vi "Error Word Bits Checker.vi"(6 "error text in":string, 8 "error in":errorcluster, 9 "number of bits":i32, 10 "start bit":i32, 11 "reserved bits in":bool[](array[boolean])=[TRUE, TRUE, TRUE, TRUE, TRUE, TRUE, TRUE, TRUE, FALSE, FALSE, FALSE, FALSE, FALSE, FALSE, FALSE, FALSE, FALSE, FALSE, FALSE, FALSE, FALSE, FALSE, FALSE, FALSE, FALSE, FALSE, FALSE, FALSE, FALSE, FALSE, FALSE, TRUE]) -> (0 "error out":errorcluster, 3 "reserved bits out":bool[](array[boolean]))   [LabVIEW 2020, in "ARINC 429 Import.lvlib"]
uses:
  ARINC 429 Import.lvlib
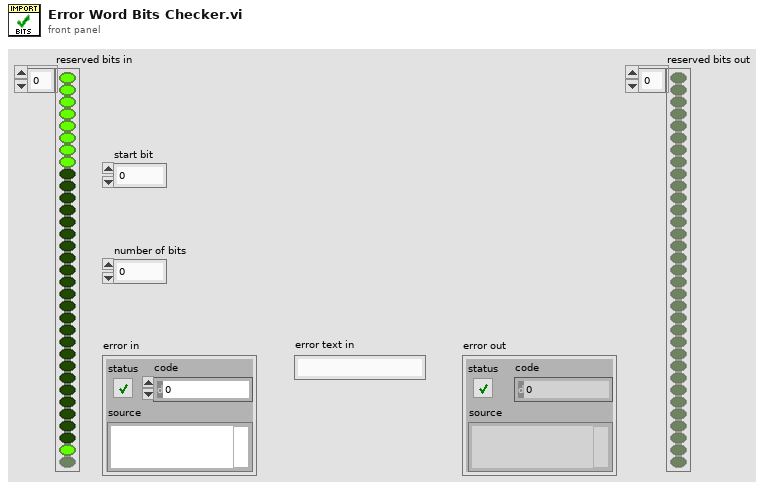
[diagram p1: front panel]
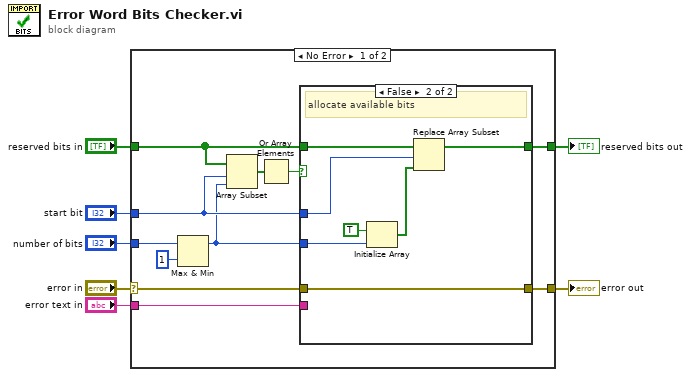
[diagram p0: block diagram]
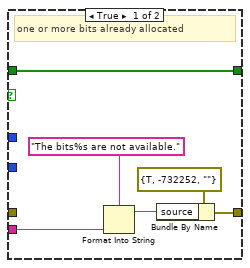
[diagram p2: hidden frame]
diagram:
  n1 = case shown="No Error" "error in" {
    selector: "error in" -> [w14 w33]
    tunnel: "start bit" -> [w18 _]
    tunnel: "number of bits" -> [w17 _]
    tunnel: [w15 w33] -> w4
    tunnel: "error text in" -> [w16 _]
    tunnel: "reserved bits in" -> [w13 w32]
    tunnel: [w8 w32] -> w1
    frame No Error {
      n2 = Max & Min(x=w17, y=1) -> (max(x,y)=w9:i32)  [unwired: 1 out]
      n3 = Array Subset(array=w13, index=w18, length=w9) -> (w12:bool[])
      n4 = Or Array Elements(Boolean array=w12) -> (logical OR=w11:bool)
      n5 = case shown="False" w11 {
        tunnel: [w24 w31] -> w8
        tunnel: w13 -> [w24 w30]
        tunnel: w9 -> [_ w29]
        tunnel: w18 -> [_ w26]
        tunnel: w16 -> [w20 _]
        tunnel: [w19 w25] -> w15
        tunnel: w14 -> [_ w25]
        frame True {
          # "one or more bits already allocated"
          n6 = Format Into String(format string="The bits%s are not available." ("source"), w20) -> (resulting string=w23:string)  [unwired: 2 in, 1 out]
          n7 = Bundle By Name(cluster=errorcluster {"status"=TRUE, "code"=-732252, "source"=""} ("error constant"), "source"=w23) -> (w19:errorcluster)
        }
        frame False {
          # "allocate available bits"
          n8 = Initialize Array(TRUE, w29) -> (w27:bool[])
          n9 = Replace Array Subset(array=w30, new element=w27, index=w26) -> (w31:bool[])
        }
      }
    }
    frame Error {
    }
  }
  "error out" <- w4
  "reserved bits out" <- w1
